vi "configure.vi"(8 "error in (no error)":errorcluster, 11 "LightSourceDL090903Laser in":refnum<class "LightSourceDL090903Laser.lvclass">) -> (0 "error out":errorcluster, 3 "LightSourceDL090903Laser out":refnum<class "LightSourceDL090903Laser.lvclass">)   [LabVIEW 2010, in "LightSourceDL090903Laser.lvclass"]
doc: "The dynamic dispatch version of this VI loads and displays the configuration file associated with the plug-in object. The user modify and save the configuration data."
uses:
  LightSourceDL090903Laser.lvclass
  type_enum.ctl
  laser_medium_enum.ctl
  pulse_enum.ctl
  common/clusters/plugin_specification.ctl
  LightSourceDL090903Laser.lvclass/LightSourceDL090903Laser.ctl
  common/classes/GenericComponent/GenericComponent/GenericComponent.lvclass
panel:
  in  "Pump laser":string(combo)
  out "LSID":string
  out "Configuration":string
  in  "cancel button":bool
  in  "save button":bool
  in  "Tunable?":bool
  in  "Frequency multiplication":dbl=1.0
  in  "Repetition rate":dbl[unit]
  in  "Pulse":T1
  in  "Laser medium":T2=enum."Unknown"
  in  "Type":T3=enum."Unknown"
  in  "Serial number":string
  in  "Model":string
  in  "Manufacturer":string
  # "Configure LightSourceDL090903Laser"
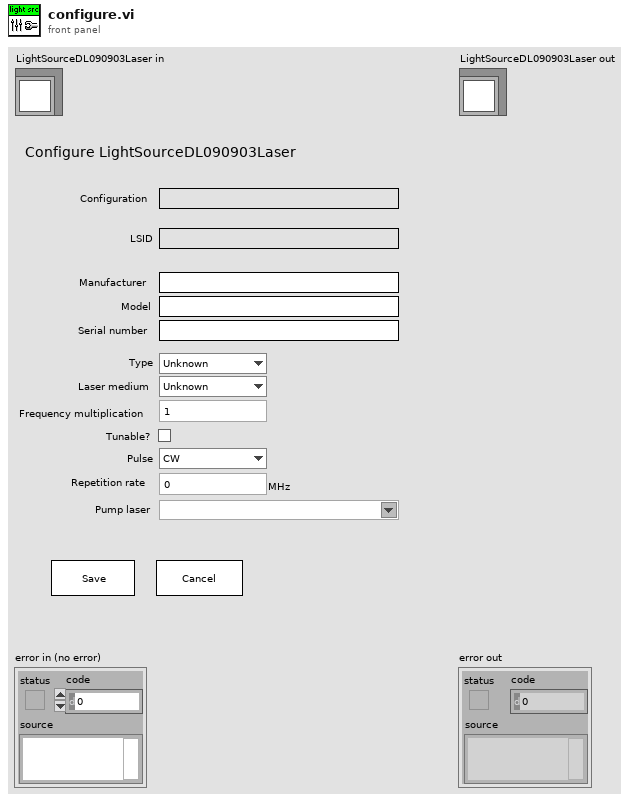
[diagram p1: front panel]
types:
  T1 = typedef "LightSourceDL090903Laser.lvclass/pulse_enum.ctl" = enum16{"CW", "Single", "QSwitched", "Repetitive", "ModeLocked"}
  T2 = typedef "LightSourceDL090903Laser.lvclass/laser_medium_enum.ctl" = enum16{"Cu", "Ag", "ArFl", "ArCl", "KrFl", "XeFl", "XeCl", "XeBr", "N", "Ar", "Kr", "Xe", "HeNe", "HeCd", "CO", "CO2", "H2O", "HFl", "NdGlass", "NdYAG", "ErGlass", "ErYAG", "HoYLF", "HoYAG", "Ruby", "TiSapphire", "Alexandrite", "Rhodamine6G", "CoumarineC30", "GaAs", "GaAlAs", "EMinus", "Unknown"}
  T3 = typedef "LightSourceDL090903Laser.lvclass/type_enum.ctl" = enum16{"Excimer", "Gas", "MetalVapor", "SolidState", "Dye", "Semiconductor", "FreeElectron", "Unknown"}
  T4 = typedef "plugin_specification.ctl" = cluster{"class path":string, "configuration":string, "label":string, "settings name":string}
  T5 = enum8{"Enabled", "Disabled", "Disabled and Grayed Out"}
  T6 = typedef "LSID_cluster.ctl" = cluster{"identifier":string, "revision":i32}
  T7 = typedef "LightSourceDL090903Laser.lvclass/config_data_cluster.ctl" = cluster{"LSID":T6, "manufacturer specification":T8, "type":T3, "laser medium":T2, "frequency multiplication":dbl, "tuneable?":bool, "pulse":T1, "repetition rate":dbl[unit], "pump laser configuration":string}
  T8 = typedef "manufacturer_specification_cluster.ctl" = cluster{"manufacturer":string, "model":string, "serial number":string, "lot number":string}
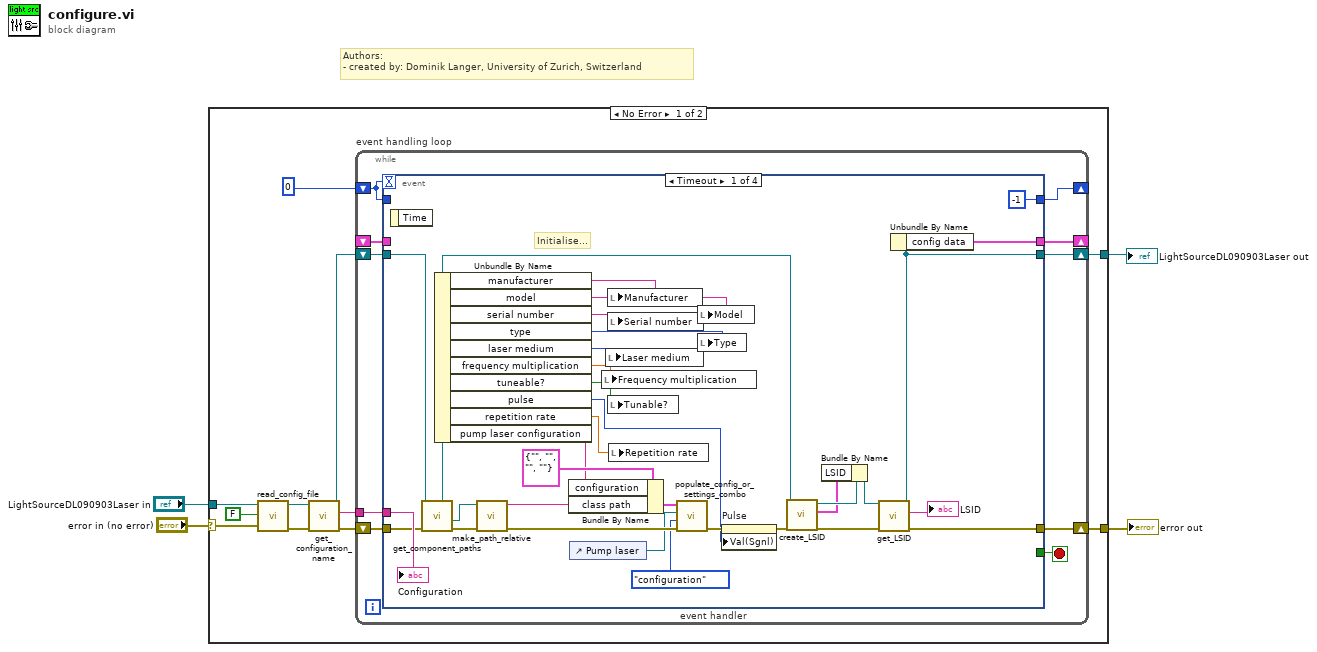
[diagram p0: block diagram]
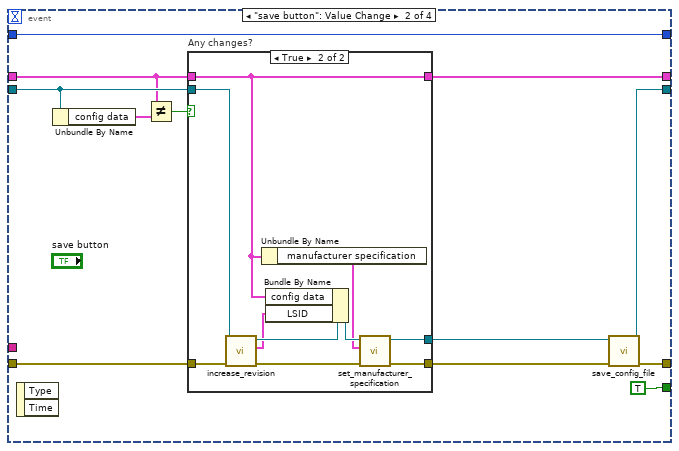
[diagram p2: hidden frame]
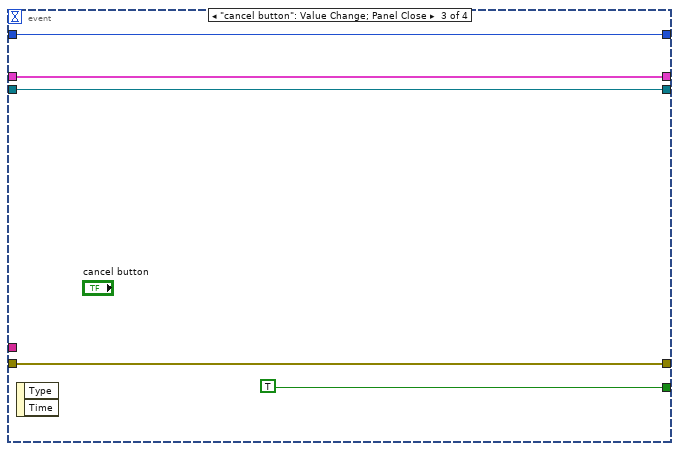
[diagram p4: hidden frame]
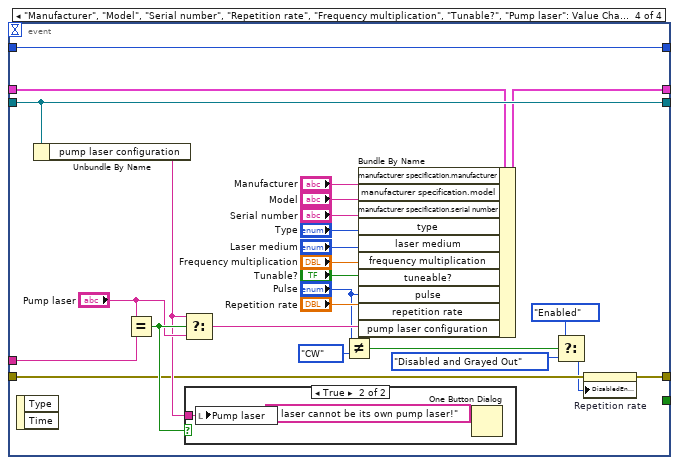
[diagram p5: hidden frame]
diagram:
  # "Authors: \n- created by: Dominik Langer, University of Zurich, Switzerland"
  n1 = case shown="No Error" "error in (no error)" {
    selector: "error in (no error)" -> [w13 w116]
    tunnel: "LightSourceDL090903Laser in" -> [w11 w117]
    tunnel: [w15 w117] -> w2
    tunnel: [w14 w116] -> w1
    frame No Error {
      n2 = call-dynamic "read_config_file.vi"("error in (no error)"=w13, "force load?"=FALSE, "GenericPlugin in"=w11) -> ("error out"=w9:errorcluster, "GenericPlugin out"=w7:refnum<class "LightSourceDL090903Laser.lvclass">)  [unwired: 7 in]
      n3 = call "get_configuration_name.vi"("error in (no error)"=w9, "GenericPlugin.lvclass in"=w7) -> ("error out"=w8:errorcluster, "configuration name"=w5:string, "GenericPlugin.lvclass out"=w6:refnum<class "LightSourceDL090903Laser.lvclass">)  [unwired: 7 in]
      n4 = while "event handling loop" {
        shift-right: [w22] -> w14
        shift-left: w8 -> [w25]
        shift-right: [w23] -> w15
        shift-left: w6 -> [w24]
        shift-right: [w19] -> _
        shift-left: 0 -> [w20]
        shift-right: [w18] -> _
        shift-left: _ -> [w17]
        tunnel: w5 -> [w16]
        stop <- w21 stop-if-true
        n5 = event "event handler" shown="[0] Timeout" {
          selector: _ -> [_ _ _ _]
          dyn-events: _ -> [_ _ _ _]
          timeout: w20 -> [_ _ _ _]
          tunnel: w25 -> [w34 w66 w87 w97]
          tunnel: w24 -> [w33 w64 w88 w91]
          tunnel: [w40 w70 w88 w91] -> w23
          tunnel: [w45 w69 w87 w96] -> w22
          tunnel: [_ TRUE TRUE _] -> w21
          tunnel: [-1 w67 w85 w105] -> w19
          tunnel: w20 -> [_ w67 w85 w105]
          tunnel: [w39 w60 w84 w89] -> w18
          tunnel: w17 -> [_ w61 w84 w90]
          tunnel: w16 -> [w46 _ _ w102]
          event Timeout {
            # "Initialise..."
            n6 = event-data() -> ()  [unwired: 1 in, 1 out]
            n7 = call-dynamic "get_component_paths.vi"("error in (no error)"=w34, "GenericComponent in"=w33) -> ("error out"=w31:errorcluster, "component class path"=w30:path, "GenericComponent out"=w32:refnum<class "LightSourceDL090903Laser.lvclass">)  [unwired: 4 in, 3 out]
            n8 = Unbundle By Name(w32) -> ("manufacturer"=w58:string, "model"=w57:string, "serial number"=w56:string, "type"=w55:T3, "laser medium"=w54:T2, "frequency multiplication"=w53:dbl, "tuneable?"=w52:bool, "pulse"=w43:T1, "repetition rate"=w51:dbl[unit], "pump laser configuration"=w47:string)
            n9 = call "make_path_relative.vi"("error in (no error)"=w31, "absolute path"=w30) -> ("error out"=w28:errorcluster, "relative path"=w29:string)  [unwired: 8 in]
            n10 = Bundle By Name(cluster=T4 {"class path"="", "configuration"="", "label"="", "settings name"=""} ("plug-in specification"), "configuration"=w47, "class path"=w29) -> (w35:T4)
            n11 = control-ref of="Pump laser"() -> (w27:refnum<vi>)
            n12 = local write "Frequency multiplication"(w53) -> ()
            n13 = local write "Laser medium"(w54) -> ()
            n14 = local write "Manufacturer"(w58) -> ()
            n15 = local write "Serial number"(w56) -> ()
            n16 = local write "Tunable?"(w52) -> ()
            n17 = local write "Repetition rate"(w51) -> ()
            n18 = call "populate_config_or_settings_combo.vi"("error in (no error)"=w28, "type"=enum16{"configuration", "settings"}."configuration", "combo-box reference"=w27, "plug-in specification"=w35) -> ("error out"=w44:errorcluster)  [unwired: 7 in]
            n19 = local write "Model"(w57) -> ()
            n20 = local write "Type"(w55) -> ()
            n21 = property on="Pulse" class="Enum (strict)"(error in=w44, "Val(Sgnl)"=w43) -> (error out=w42:errorcluster)  [unwired: 1 in, 1 out]
            n22 = call-dynamic "create_LSID.vi"("error in (no error)"=w42, "GenericPlugin in"=w32) -> ("error out"=w41:errorcluster, "current LSID"=w36:T6, "GenericPlugin out"=w38:refnum<class "LightSourceDL090903Laser.lvclass">)  [unwired: 7 in]
            n23 = Bundle By Name(cluster=w38, "LSID"=w36) -> (w37:refnum<class "LightSourceDL090903Laser.lvclass">)
            n24 = call-dynamic "get_LSID.vi"("error in (no error)"=w41, "GenericPlugin in"=w37) -> ("error out"=w45:errorcluster, "LSID (string)"=→"LSID":string, "GenericPlugin out"=w40:refnum<class "LightSourceDL090903Laser.lvclass">)  [unwired: 6 in, 1 out]
            n25 = Unbundle By Name(w40) -> ("config data"=w39:T7)
            "Configuration" <- w46
          }
          event "save button": Value Change {
            n26 = event-data() -> ()  [unwired: 1 in, 2 out]
            n27 = Unbundle By Name(w64) -> ("config data"=w63:T7)
            n28 = Not Equal?(x=w61, y=w63) -> (x != y?=w62:bool)
            n29 = case "Any changes?" shown="True" w62 {
              tunnel: w66 -> [w73 w83]
              tunnel: [w73 w77] -> w65
              tunnel: w64 -> [w72 w80]
              tunnel: [w72 w75] -> w59
              tunnel: w61 -> [w71 w79]
              tunnel: [w71 w79] -> w60
              frame False {
              }
              frame True {
                n30 = call-dynamic "increase_revision.vi"("error in (no error)"=w83, "GenericPlugin in"=w80) -> ("error out"=w78:errorcluster, "new LSID"=w81:T6, "GenericPlugin out"=w82:refnum<class "LightSourceDL090903Laser.lvclass">)  [unwired: 7 in]
                n31 = Unbundle By Name(w79) -> ("manufacturer specification"=w74:T8)
                n32 = Bundle By Name(cluster=w82, "config data"=w79, "LSID"=w81) -> (w76:refnum<class "LightSourceDL090903Laser.lvclass">)
                n33 = call-dynamic "set_manufacturer_specification.vi"("error in (no error)"=w78, "manufacturer specification"=w74, "GenericPlugin in"=w76) -> ("error out"=w77:errorcluster, "GenericPlugin out"=w75:refnum<class "LightSourceDL090903Laser.lvclass">)  [unwired: 7 in]
              }
            }
            n34 = call-dynamic "save_config_file.vi"("error in (no error)"=w65, "GenericPlugin in"=w59) -> ("error out"=w69:errorcluster, "GenericPlugin out"=w70:refnum<class "LightSourceDL090903Laser.lvclass">)  [unwired: 8 in]
          }
          event "cancel button": Value Change; Panel Close {
            n35 = event-data() -> ()  [unwired: 1 in, 2 out]
          }
          event "Manufacturer", "Model", "Serial number", "Repetition rate", "Frequency multiplication", "Tunable?", "Pump laser": Value Change {
            n36 = event-data() -> ()  [unwired: 1 in, 2 out]
            n37 = Unbundle By Name(w91) -> ("pump laser configuration"=w100:string)
            n38 = Equal?(x="Pump laser", y=w102) -> (x = y?=w103:bool)
            n39 = Select(t=w100, s=w103, f="Pump laser") -> (s? t:f=w104:string)
            n40 = case shown="True" w103 {
              tunnel: w100 -> [_ w114]
              frame False {
              }
              frame True {
                n41 = local write "Pump laser"(w114) -> ()
                n42 = One Button Dialog(message="A laser cannot be its own pump laser!") -> ()  [unwired: 1 in, 1 out]
              }
            }
            n43 = Not Equal?(x="Pulse", y=pulse_enum."CW") -> (x != y?=w95:bool)
            n44 = Bundle By Name(cluster=w90, "manufacturer specification.manufacturer"="Manufacturer", "manufacturer specification.model"="Model", "manufacturer specification.serial number"="Serial number", "type"="Type", "laser medium"="Laser medium", "frequency multiplication"="Frequency multiplication", "tuneable?"="Tunable?", "pulse"="Pulse", "repetition rate"="Repetition rate", "pump laser configuration"=w104) -> (w89:T7)
            n45 = Select(t=T5."Enabled" ("Disabled"), s=w95, f=T5."Disabled and Grayed Out") -> (s? t:f=w93:T5)
            n46 = property on="Repetition rate" class="DigNum (strict)"(error in=w97, "DisabledEnum"=w93) -> (error out=w96:errorcluster)  [unwired: 1 in, 1 out]
          }
        }
      }
    }
    frame Error {
    }
  }
  "error out" <- w1
  "LightSourceDL090903Laser out" <- w2
